vi "RM.forceDeleteReservation.vi"(5 "Resource Type":T1, 7 "Direction":T2, 8 "error in":errorcluster, 10 "name in bitfile":string, 11 "reservation DB in":variant) -> (0 "error out":errorcluster, 2 "found?":bool, 3 "reservation DB out":variant)   [LabVIEW 2016, in "FPGA Addon Shared.lvlib"]
uses:
  FPGA Addon Shared.lvlib
  RM.resourceDirection.ctl
  RM.resourceType.ctl
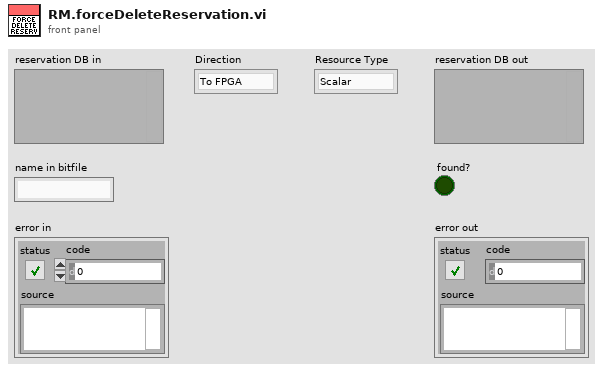
[diagram p1: front panel]
types:
  T1 = typedef "FPGA Addon Shared.lvlib/RM.resourceType.ctl" = enum16{"Scalar", "Waveform"}
  T2 = typedef "FPGA Addon Shared.lvlib/RM.resourceDirection.ctl" = enum16{"To FPGA", "From FPGA"}
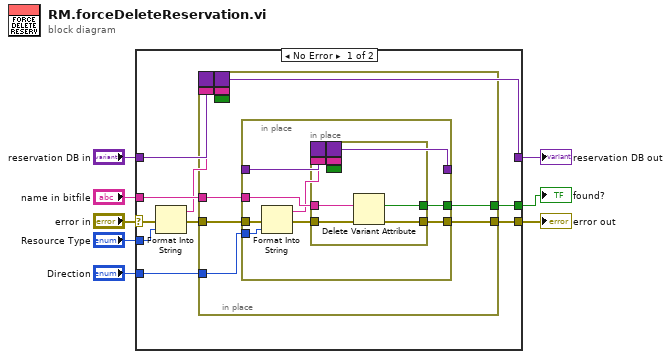
[diagram p0: block diagram]
diagram:
  n1 = case shown="No Error" "error in" {
    selector: "error in" -> [w11 w41]
    tunnel: "reservation DB in" -> [w18 w42]
    tunnel: "Direction" -> [w17 _]
    tunnel: [w16 w42] -> w1
    tunnel: "name in bitfile" -> [w15 _]
    tunnel: "Resource Type" -> [w14 _]
    tunnel: [w10 w41] -> w3
    tunnel: [w9 _] -> w2
    frame No Error {
      n2 = Format Into String(error in=w11, w14) -> (resulting string=w13:string, error out=w12:errorcluster)  [unwired: 2 in]
      n3 = in-place {
        in-place-border: w17 -> [w25]
        in-place-border: w15 -> [w22]
        in-place-border: w12 -> [w21]
        in-place-border: [w20] -> w10
        in-place-border: [w19] -> w9
        border: w18 -> [_]
        border: w13 -> [_]
        border: [_] -> w16
        border: _ -> [_]
        border: _ -> [_]
        n4 = in-place {
          in-place-border: w25 -> [w31]
          in-place-border: w24 -> [w34]
          in-place-border: [w33] -> w23
          in-place-border: w22 -> [w32]
          in-place-border: w21 -> [w29]
          in-place-border: [w27] -> w20
          in-place-border: [w26] -> w19
          n5 = Format Into String(error in=w29, w31) -> (resulting string=w30:string, error out=w28:errorcluster)  [unwired: 2 in]
          n6 = in-place {
            in-place-border: w32 -> [w36]
            in-place-border: w28 -> [w39]
            in-place-border: [w38] -> w27
            in-place-border: [w37] -> w26
            border: w34 -> [_]
            border: w30 -> [_]
            border: [_] -> w33
            border: _ -> [_]
            border: _ -> [_]
            n7 = Delete Variant Attribute(4:w39, 6:w36, 7:w35) -> (0:w38:errorcluster, 2:w37:bool, 3:w40:variant)
          }
        }
      }
    }
    frame Error {
    }
  }
  "reservation DB out" <- w1
  "error out" <- w3
  "found?" <- w2
